vi "ecg_ncs_v5.vi"() -> ()   [LabVIEW 2016]
uses:
  <instrlib>/niUSRP/niUSRP Timestamp.ctl
  C:/Program Files/National Instruments/LabVIEW 2016/examples/Instrument IO/Serial/support/Serial - Settings.ctl
  State.ctl
  <vilib>/Instr/_visa.llb/VISA Configure Serial Port (Instr).vi
  <instrlib>/niUSRP/niUSRP Write Tx Data (2D CDB).vi
  <instrlib>/niUSRP/niUSRP Fetch Rx Data (2D CDB).vi
panel:
  in  "File Name 2":string="Test"
  in  "Path 2":path=path "D:/Research/SummerFall17Spring18/CnC/NCS/EcgNcsCorrelation/Labview Codes/ECG_NCS"
  out "#Loop = #Packets Received":i32
  out "ECGsample":i16
  out "PhNcs":dbl
  out "AmpNcs":dbl
  out "AmpNcsDS":dbl
  out "PhNcsDS":dbl
  out "error IO 2":errorcluster={"status"=FALSE, "code"=-1074118647, "source"=""}
  in  "Serial Settings":T1={"baud rate"=57600, "data bits"=8, "parity"=enum."None", "stop bits"=10, "flow control"=0} {"flow control" items=["None"=0, "XON/XOFF"=1, "RTS/CTS"=2, "DTR/DSR"=4]; "stop bits" items=["1.0"=10, "1.5"=15, "2.0"=20]; "data bits" min=5 max=8 step=1; "baud rate" items=["75"=75, "110"=110, "134"=134, "150"=150, "300"=300, "600"=600, "1200"=1200, "1800"=1800, "2400"=2400, "4800"=4800, "7200"=7200, "9600"=9600, "14400"=14400, "19200"=19200, "28800"=28800, "38400"=38400, "56000"=56000, "57600"=57600, "115200"=115200, "128000"=128000, "230400"=230400]}
  in  "VISA resource name":refnum<visa-resource-name>="bmd101"
  out "ECG":i16(graph)
  in  "byte count":u32=1
  out "Coerced Rx IQ Rate":dbl
  in  "Sampling Rate":i32=500
  out "Gain":dbl=-15.0
  out "Bandwidth":dbl=56000000.0
  out "Coerced Carrier Frequency":dbl=2000000000.0 format="%#.17g"
  out "Coerced Tx IQ rate":dbl=1000000.0
  out "error IO":errorcluster={"status"=FALSE, "code"=-1074118647, "source"=""}
  in  "Rx Number of Samples":i32=10000
  in  "Tab Control 2":enum32{"NI-294x/295x", "NI-2900/2901"}(tab)=enum."NI-2900/2901"
  in  "Rx carrier frequency [Hz]":dbl=2000000000.0 format="%#_6p"
  in  "Tx carrier frequency [Hz]":dbl=1000000000.0 format="%#_6p"
  in  "Start Trigger Time":T2={"whole seconds"=1, "fractional seconds"=0.0}
  in  "Tab Control":T3(tab)
  out "NCS tag Amp":dbl[](graph)=[0.011967714738528729, 0.012021355192189592, 0.012015275039596582, 0.011969166030167903, 0.011958890166168242, 0.012007893820858737, 0.012022893722444085, 0.011978222225113794, 0.011969989939463181, 0.012003099640895068]
  out "NCS tag Phase":dbl[](graph)=[0.011967714738528729, 0.012021355192189592, 0.012015275039596582, 0.011969166030167903, 0.011958890166168242, 0.012007893820858737, 0.012022893722444085, 0.011978222225113794, 0.011969989939463181, 0.012003099640895068]
  out "Tag Amp":dbl[](graph)
  out "Tag Phase":dbl[](graph)
  out "Tx Waveform Graph":waveform(dbl)[](graph)
  in  "Stop":bool
  in  "Channel 0\nTone Amplitude":dbl=0.707 step=0.05 format="%#.6g"
  in  "Channel 0 \nTone Frequency":dbl=5000.0 format="%#_6p"
  in  "Tx Waveform Size":dbl=2000.0
  in  "Device Name":refnum<k15>="MyB200"
  in  "Tx Gain":dbl=28.0 format="%#_6f"
  in  "Tx IQ Rate":dbl=1000000.0 format="%#_6p"
  in  "Rx Gain":dbl=32.0 format="%#_6f"
  in  "Rx IQ Rate":dbl=1000000.0 format="%#_6p"
  # "Rx Settings"
  # "Tx Settings"
  # "Note that on the NI-2900 and NI-2901, both Rx channels share an LO and both Tx channels share an LO. However, on the NI-294x/295x devices, Rx and Tx of channel 0 share an LO and Rx and Tx of channel 1 share an LO."
  # "Rx: Number of samples should be 1e6/512 in one loop."
  # "This Tx graph should always have end and start tied up since this is being sent in a loop continuously. Otherwise phase jumps will be noticed."
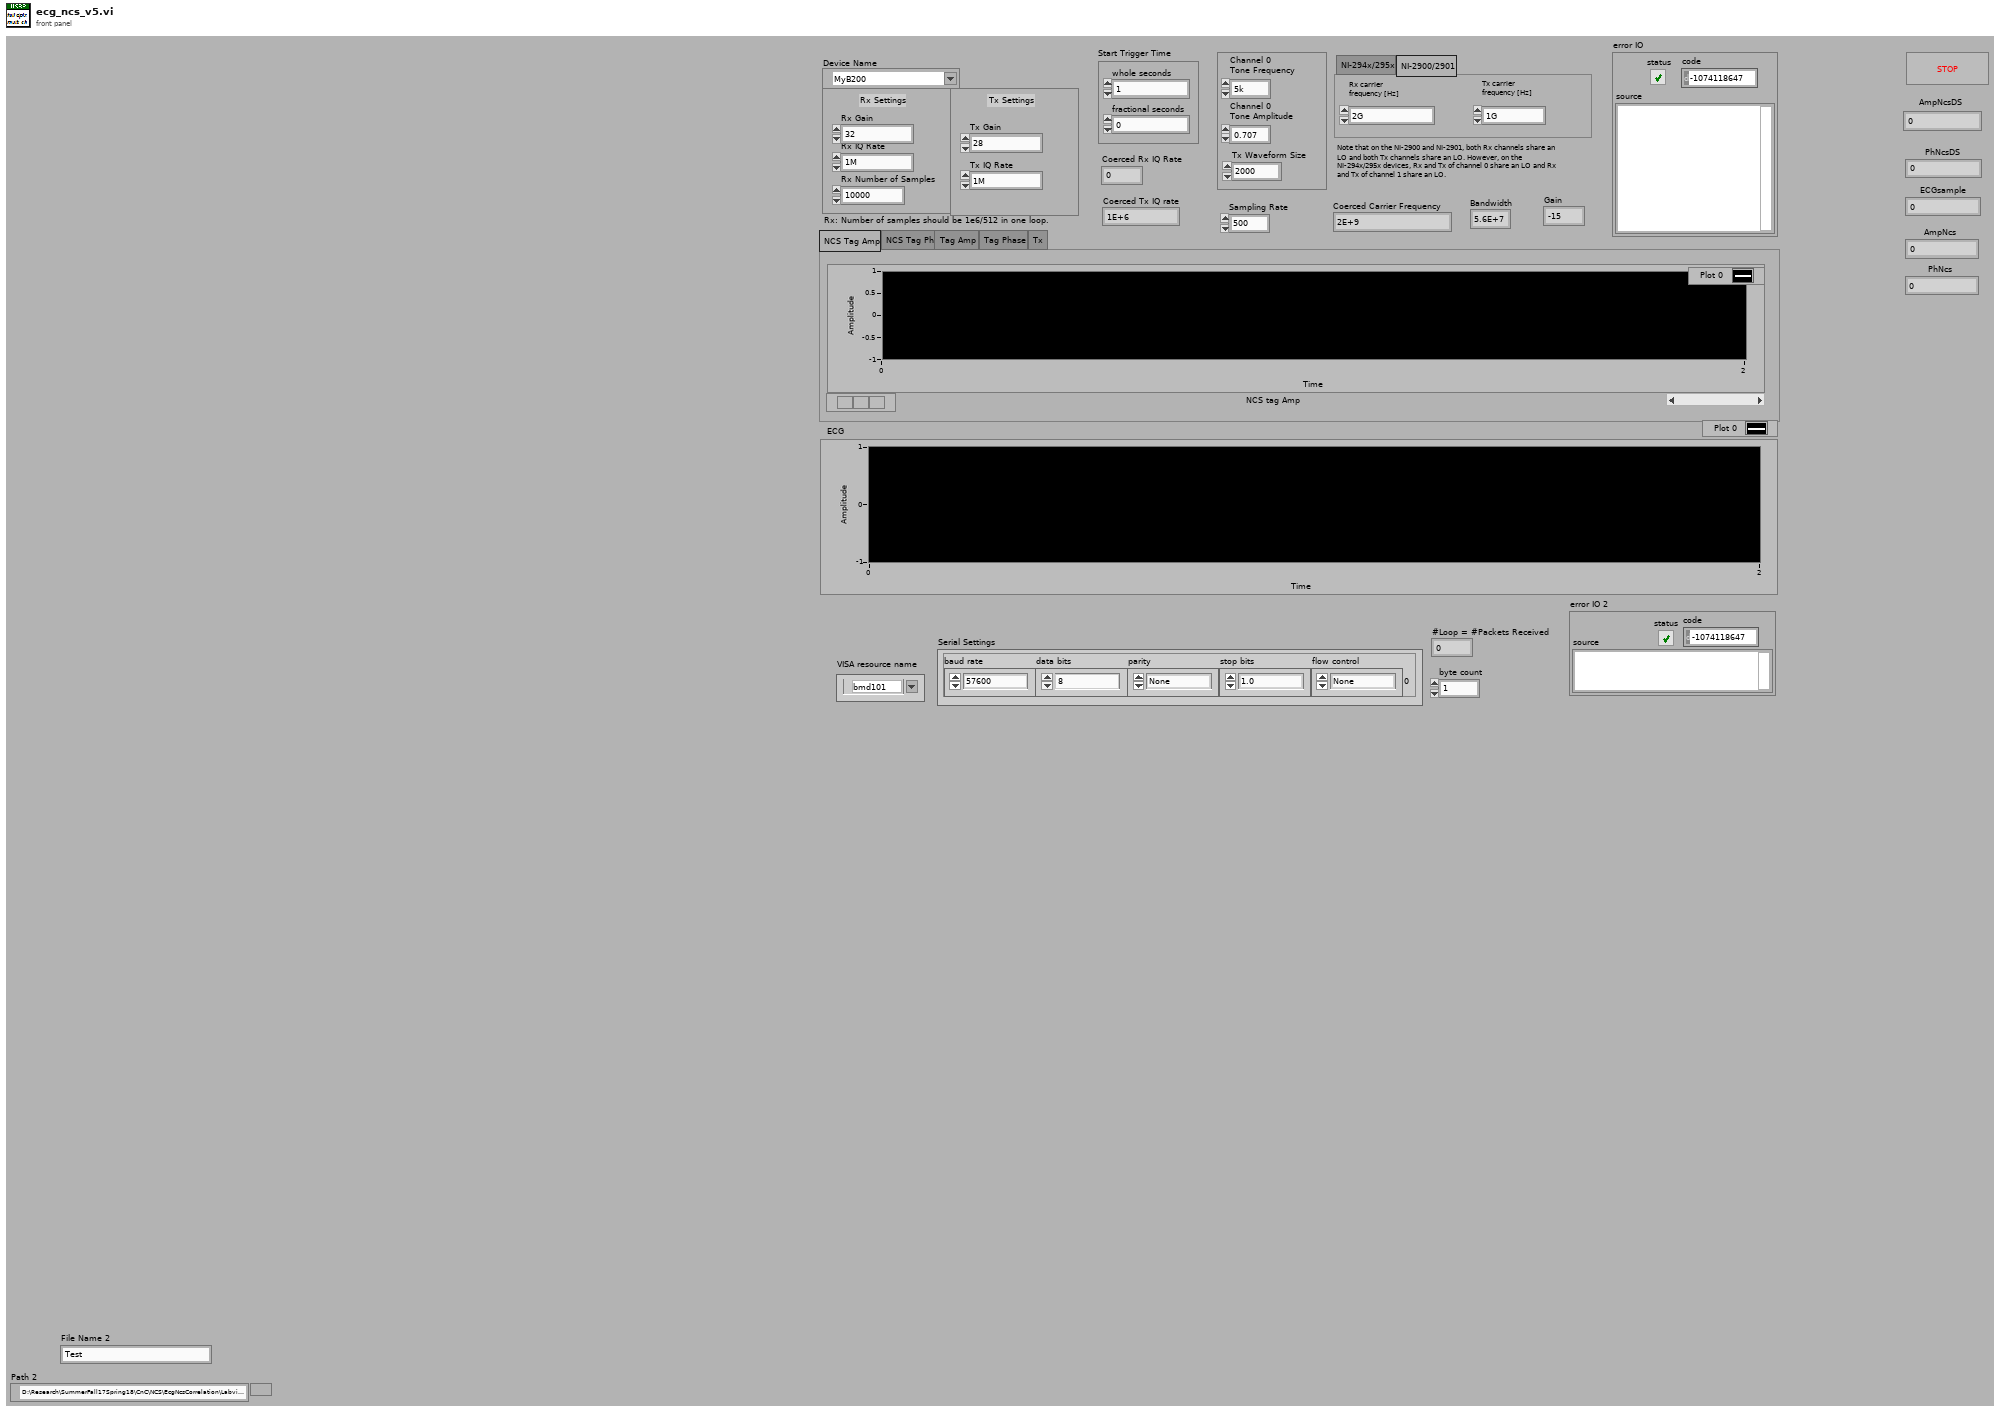
[diagram p1: front panel]
types:
  T1 = typedef "Serial - Settings.ctl" = cluster{"baud rate":u32, "data bits":u16, "parity":enum16{"None", "Odd", "Even", "Mark", "Space"}, "stop bits":u16, "flow control":u16}
  T2 = typedef "niUSRP Timestamp.ctl" = cluster{"whole seconds":u64, "fractional seconds":dbl}
  T3 = enum32{"NCS Tag Amp", "NCS Tag Ph", "Tag Amp", "Tag Phase", "Tx"}
  T4 = typedef "State.ctl" = enum16{"Initialize", "get byte", "check", "packet received", "packet approved"}
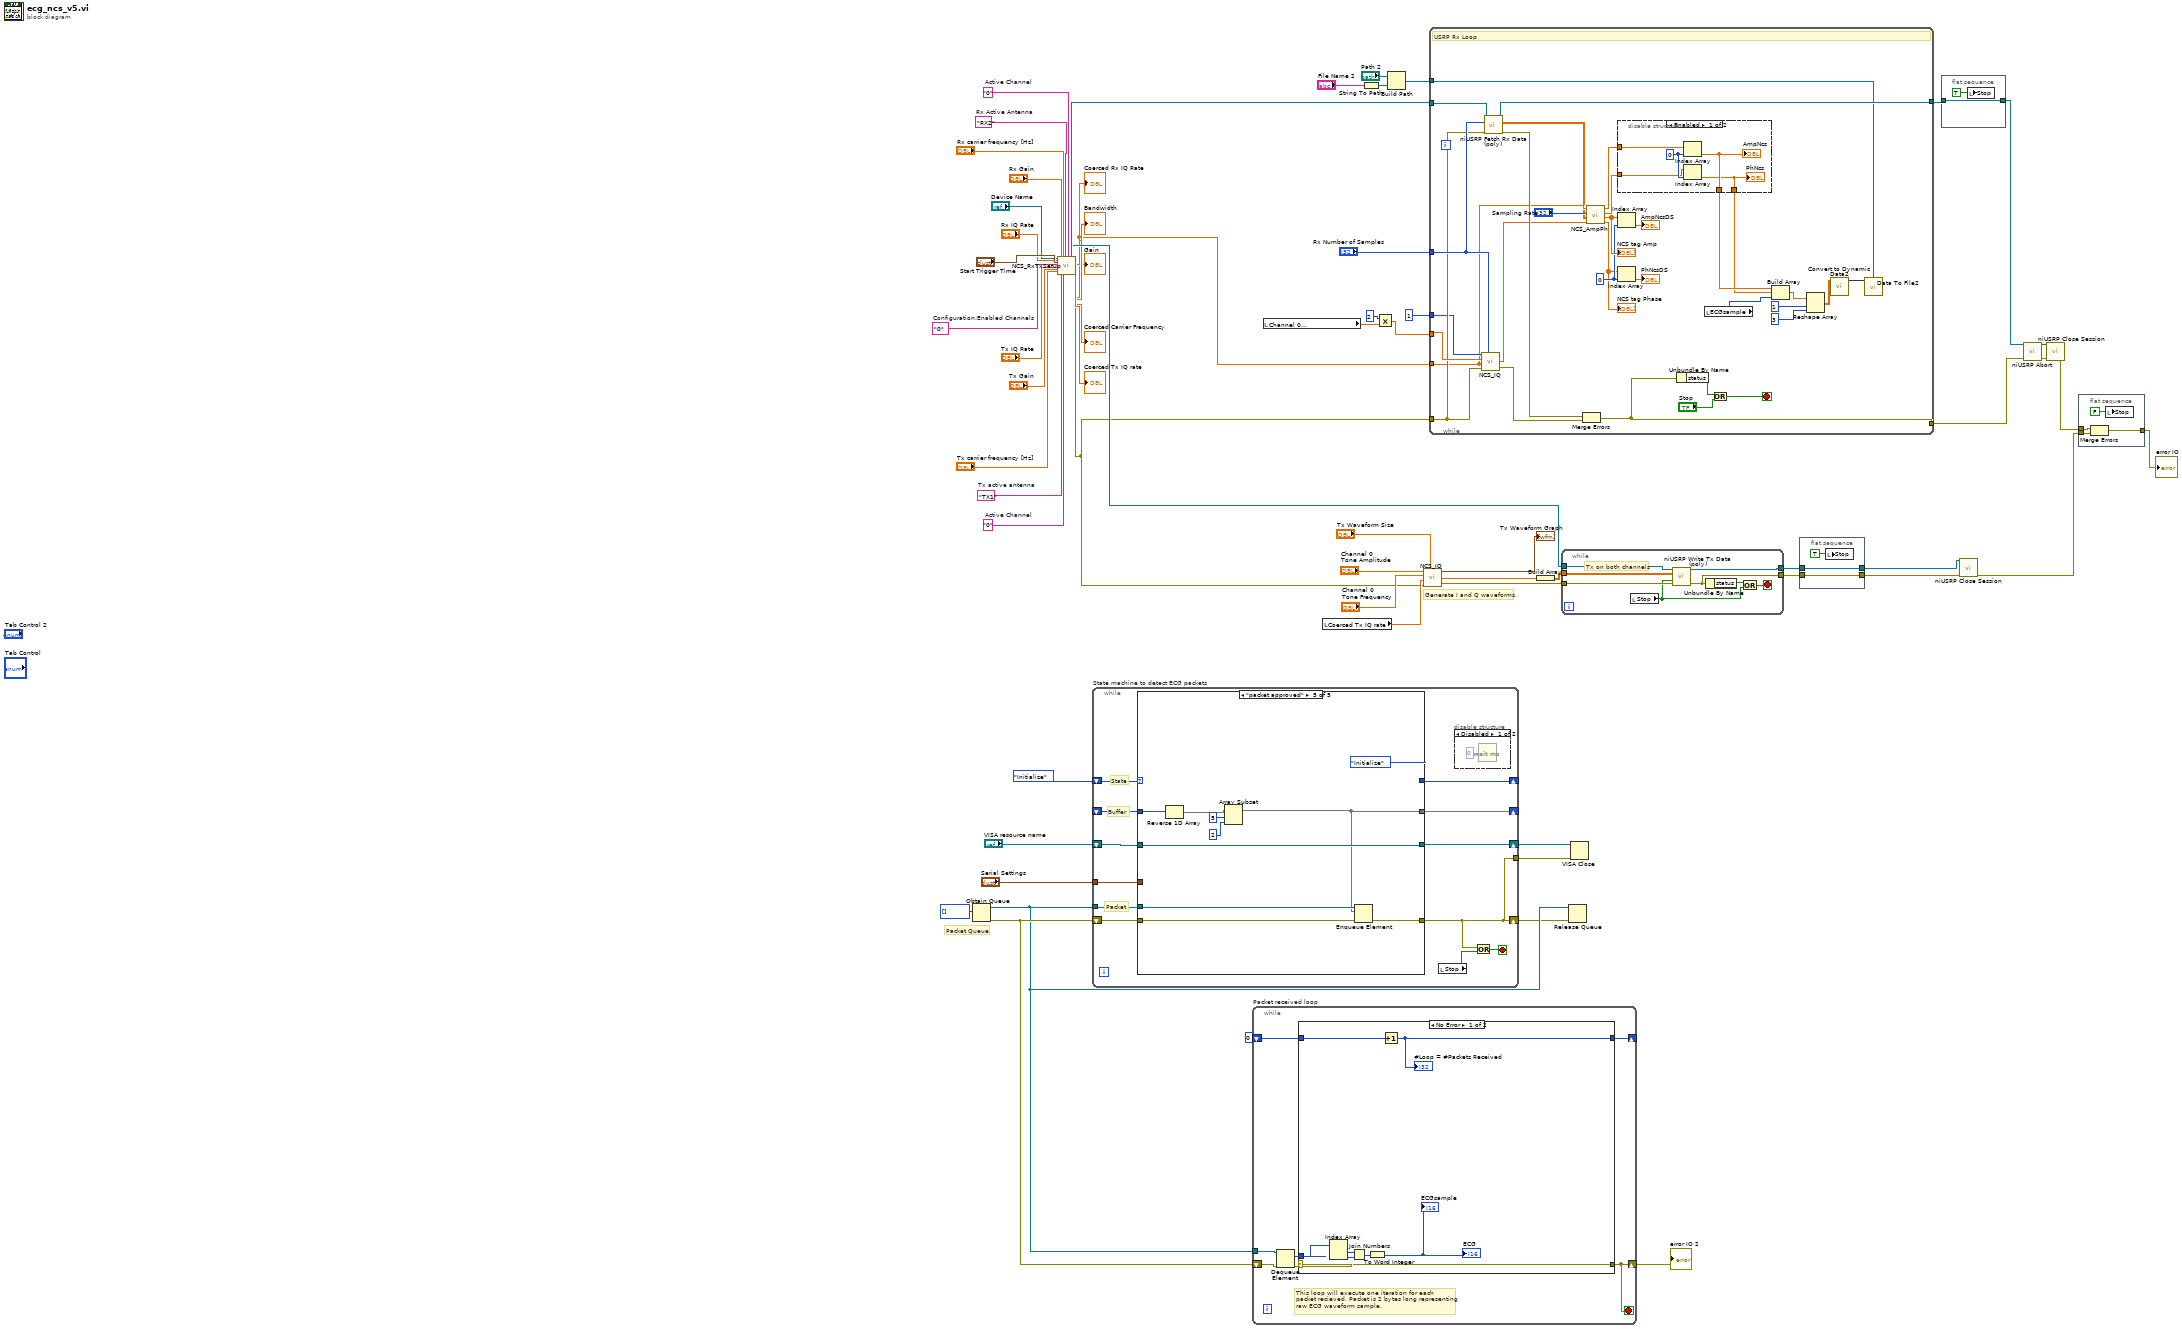
[diagram p0: block diagram]
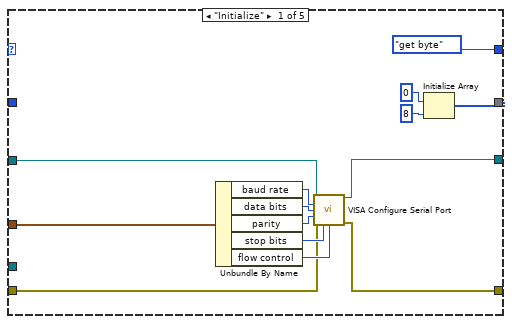
[diagram p4: hidden frame]
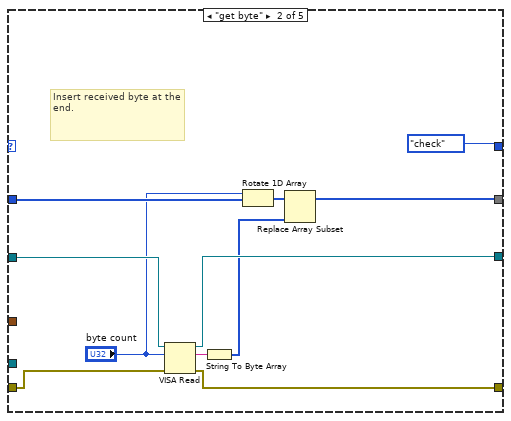
[diagram p5: hidden frame]
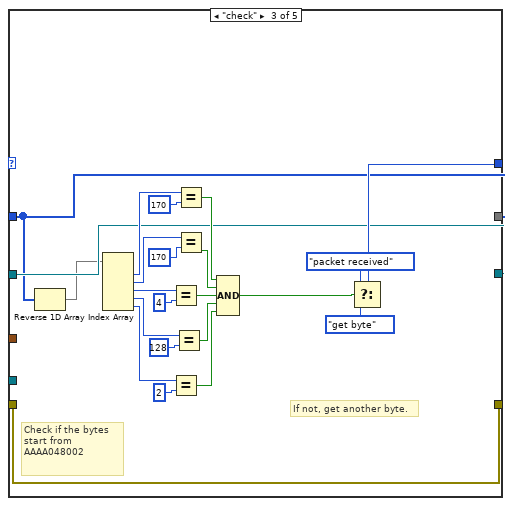
[diagram p6: hidden frame]
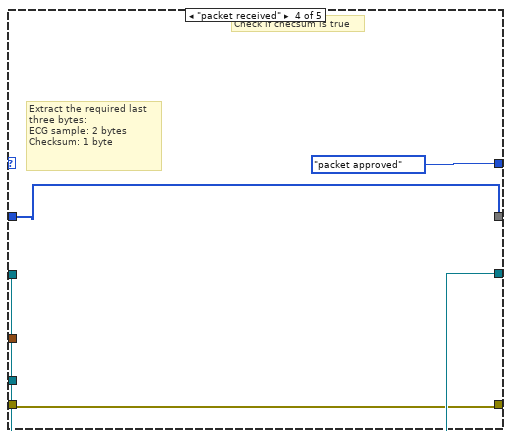
[diagram p7: hidden frame]
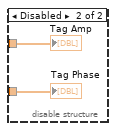
[diagram p8: hidden frame]
diagram:
  w17 = "0"  # Active Channel
  w18 = "0"  # Active Channel
  w53 = "RX2"  # Rx Active Antenna
  w49 = "TX1"  # Tx active antenna
  w35 = "0"  # Configuration:Enabled Channels
  # "Packet Queue"
  # "Generate I and Q waveforms."
  n1 = Obtain Queue(element data type=u8[] []) -> (queue out=w12:refnum<queue>, error out=w13:errorcluster)  [unwired: 4 in, 1 out]
  n2 = call "NCS_RxTxSetup.vi"("IVI Refnum in"="Device Name", "Rx IQ Rate"="Rx IQ Rate", "Start Trigger Time"="Start Trigger Time", "Configuration:Enabled Channels"=w35, "Tx IQ Rate"="Tx IQ Rate", "Tx Gain"="Tx Gain", "Tx carrier frequency [Hz]"="Tx carrier frequency [Hz]", "Rx Gain"="Rx Gain", "Tx active antenna"=w49, "Rx carrier frequency [Hz]"="Rx carrier frequency [Hz]", "Active Channel"=w17, "Rx Active Antenna"=w53, "Active Channel 2"=w18) -> ("session handle out"=w60:refnum<k15>, "IVI Refnum out"=w61:refnum<k15>, "Coerced Rx IQ Rate"=w16:dbl, "Bandwidth"=→"Bandwidth":dbl, "Gain"=→"Gain":dbl, "Carrier Frequency"=→"Coerced Carrier Frequency":dbl, "IQ Rate 2"=→"Coerced Tx IQ rate":dbl, "error out"=w28:errorcluster)  [unwired: 7 in]
  "Coerced Rx IQ Rate" <- w16
  n3 = while "State machine to detect ECG packets" {
    shift-right: [w64] -> w7
    shift-left: w13 -> [w70]
    shift-right: [w73] -> _
    shift-left: State."Initialize" ("State") -> [w72]
    shift-right: [w69] -> _
    shift-left: _ -> [w71]
    tunnel: w12 -> [w68]
    shift-right: [w67] -> w8
    shift-left: "VISA resource name" -> [w66]
    tunnel: "Serial Settings" -> [w65]
    tunnel: [w64] -> w6
    stop <- w63 stop-if-true
    # "State"
    # "Buffer"
    # "Packet"
    n4 = case shown="\"packet approved\"" w72 {
      tunnel: [w85 w97 w101 w124 w127] -> w69
      tunnel: [State."get byte" ("State") State."check" ("f") w121 State."packet approved" ("State") State."Initialize" ("State")] -> w73
      tunnel: w71 -> [_ w90 w101 w124 w129]
      tunnel: w70 -> [w79 w94 w122 w125 w132]
      tunnel: [w78 w93 w122 w125 w131] -> w64
      tunnel: w68 -> [_ _ _ _ w133]
      tunnel: [w77 w95 w102 w126 w130] -> w67
      tunnel: w66 -> [w76 w96 w102 w126 w130]
      tunnel: w65 -> [w75 _ _ _ _]
      frame "Initialize" {
        n5 = Unbundle By Name(w75) -> ("baud rate"=w84:u32, "data bits"=w83:u16, "parity"=w82:enum16{"None", "Odd", "Even", "Mark", "Space"}, "stop bits"=w81:u16, "flow control"=w80:u16)
        n6 = call-poly "VISA Configure Serial Port"("VISA resource name"=w76, "baud rate (9600)"=w84, "data bits (8)"=w83, "parity (0:none)"=w82, "error in (no error)"=w79, "stop bits (10: 1 bit)"=w81, "flow control (0:none)"=w80) -> ("VISA resource name out"=w77:refnum<visa-resource-name>, "error out"=w78:errorcluster)  [unwired: 3 in, 4 out]
        n7 = Initialize Array(u8 0, 8 ("dimension size")) -> (w85:u8[])
      }
      frame "get byte" {
        # "Insert received byte at the end."
        n8 = VISA Read(VISA resource name=w96, byte count="byte count", error in (no error)=w94) -> (VISA resource name out=w95:refnum<visa-resource-name>, read buffer=w92:string, error out=w93:errorcluster)  [unwired: 1 out]
        n9 = String To Byte Array(string=w92) -> (unsigned byte array=w91:u8[])
        n10 = Rotate 1D Array(1:w90, 2:"byte count") -> (0:w98:u8[])
        n11 = Replace Array Subset(array=w98, new element=w91) -> (w97:u8[])  [unwired: 1 in]
      }
      frame "check" {
        # "If not, get another byte."
        # "Check if the bytes start from AAAA048002"
        n12 = Reverse 1D Array(array=w101) -> (reversed array=w100:u8[])
        n13 = Index Array(array=w100) -> (element #1=w108:u8, element #2=w107:u8, element #3=w106:u8, element #4=w105:u8, element #5=w104:u8)  [unwired: 5 in]
        n14 = Equal?(x=w106, y=u8 4 ("element")) -> (x = y?=w111:bool)
        n15 = Equal?(x=w104, y=u8 2 ("element")) -> (x = y?=w109:bool)
        n16 = Equal?(x=w105, y=u8 128 ("element")) -> (x = y?=w110:bool)
        n17 = Equal?(x=w108, y=u8 170 ("element")) -> (x = y?=w113:bool)
        n18 = Equal?(x=w107, y=u8 170 ("element")) -> (x = y?=w112:bool)
        n19 = Compound Arithmetic op=AND(w113, w112, w111, w110, w109) -> (w103:bool)
        n20 = Select(t=State."packet received" ("f"), s=w103, f=State."get byte") -> (s? t:f=w121:T4)
      }
      frame "packet received" {
        # "Check if checsum is true"
        # "Extract the required last three bytes: \nECG sample: 2 bytes\nChecksum: 1 byte"
      }
      frame "packet approved" {
        n21 = Reverse 1D Array(array=w129) -> (reversed array=w128:u8[])
        n22 = Array Subset(array=w128, index=5, length=2 ("index")) -> (w127:u8[])
        n23 = Enqueue Element(queue=w133, element=w127, error in (no error)=w132) -> (error out=w131:errorcluster)  [unwired: 1 in, 2 out]
      }
    }
    n24 = local read "Stop"() -> (w62:bool)
    n25 = disable-structure shown="Disabled" {
      frame Disabled {
        n26 = Wait (ms)(milliseconds to wait=u32 0) -> ()  [unwired: 1 out]
      }
      frame Enabled {
      }
    }
    n27 = Or(x=w64, y=w62) -> (x .or. y?=w63:bool)
  }
  n28 = while "Packet received loop" {
    shift-right: [w139] -> w9
    shift-left: w13 -> [w143]
    tunnel: w12 -> [w142]
    shift-right: [w137] -> _
    shift-left: 0 -> [w138]
    stop <- w139 stop-if-true
    # "This loop will execute one iteration for each\npacket recieved. Packet is 2 bytes long representing \nraw ECG waveform sample."
    n29 = Dequeue Element(queue=w142, error in (no error)=w143) -> (element=w141:u8[], error out=w140:errorcluster)  [unwired: 1 in, 2 out]
    n30 = case shown="No Error" w140 {
      selector: w140 -> [w145 w153]
      tunnel: w141 -> [w151 _]
      tunnel: [w145 w153] -> w139
      tunnel: w138 -> [w147 w152]
      tunnel: [w146 w152] -> w137
      frame No Error {
        n31 = Index Array(array=w151) -> (element #1=w150:u8, element #2=w149:u8)  [unwired: 2 in]
        n32 = Join Numbers(hi=w150, lo=w149) -> ((hi.lo)=w148:u16)
        n33 = To Word Integer(number=w148) -> (16bit integer=→"ECG" →"ECGsample":i16)
        n34 = Increment(x=w147) -> (x+1=w146:i32)
        "#Loop = #Packets Received" <- w146
      }
      frame Error {
      }
    }
  }
  "error IO 2" <- w9
  n35 = local read "Channel 0 \nTone Frequency"() -> (w34:dbl)
  n36 = local read "Coerced Tx IQ rate"() -> (w29:dbl)
  n37 = String To Path(string="File Name 2") -> (path=w4:path)
  n38 = Multiply(x=2, y=w34) -> (x*y=w33:dbl)
  n39 = Build Path(base path="Path 2", name or relative path=w4) -> (appended path=w1:path)
  n40 = call "NCS_IQ.vi"("Tone Amplitude"="Channel 0\nTone Amplitude", "Waveform Size"="Tx Waveform Size", "Tone Frequency"="Channel 0 \nTone Frequency", "Coerced IQ rate"=w29, "error in (no error)"=w28) -> ("IQ waveform"=→"Tx Waveform Graph":waveform(dbl)[], "IQ waveform array"=w26:cdb[], "error out"=w27:errorcluster)  [unwired: 1 in]
  n41 = while {
    tunnel: w61 -> [w185]
    tunnel: w28 -> [w178]
    tunnel: [w184] -> w45
    tunnel: "Rx Number of Samples" -> [w180]
    tunnel: w16 -> [w174]
    tunnel: [w175] -> w37
    tunnel: w33 -> [w179]
    tunnel: 1 -> [w176]
    tunnel: w1 -> [w154]
    stop <- w181 stop-if-true
    w166 = 0
    # "USRP Rx Loop"
    n42 = call "NCS_IQ.vi"("Tone Amplitude"=w176, "Waveform Size"=w180, "Tone Frequency"=w179, "Coerced IQ rate"=w174, "error in (no error)"=w178) -> ("IQ waveform array"=w171:cdb[], "error out"=w177:errorcluster)  [unwired: 1 in, 1 out]
    n43 = call-poly <instrlib>:"niUSRP Fetch Rx Data (poly).vi"("session handle"=w185, "number of samples"=w180, "error in (no error)"=w178) -> ("session handle out"=w184:refnum<k15>, "data"=w172:cdb[][], "error out"=w182:errorcluster)  [unwired: 9 in, 1 out]
    n44 = Merge Errors(w182, w177) -> (w175:errorcluster)
    n45 = call "NCS_AmpPh.vi"("IQ"=w171, "data"=w172, "Sampling Rate"="Sampling Rate", "Coerced Rx IQ Rate"=w174) -> ("Phase DownSampled"=w165:dbl[], "Amp DownSampled"=w167:dbl[], "Phase"=w169:dbl[], "Amplitude"=w170:dbl[])  [unwired: 4 in]
    "NCS tag Amp" <- w167
    "NCS tag Phase" <- w165
    n46 = disable-structure shown="Enabled" {
      disable-tunnel: w170 -> [w189 w192]
      disable-tunnel: w169 -> [w188 w191]
      disable-tunnel: [w187 _] -> w156
      disable-tunnel: [w186 _] -> w155
      frame Enabled {
        w190 = 0
        n47 = Index Array(array=w189, index=w190) -> (element=w187:dbl)
        "AmpNcs" <- w187
        n48 = Index Array(array=w188, index=w190) -> (element=w186:dbl)
        "PhNcs" <- w186
      }
      frame Disabled {
        "Tag Amp" <- w192
        "Tag Phase" <- w191
      }
    }
    n49 = Index Array(array=w167, index=w166) -> (element=→"AmpNcsDS":dbl)
    n50 = Index Array(array=w165, index=w166) -> (element=→"PhNcsDS":dbl)
    n51 = Unbundle By Name(w175) -> ("status"=w183:bool)
    n52 = local read "ECGsample"() -> (w157:i16)
    n53 = Or(x=w183, y="Stop") -> (x .or. y?=w181:bool)
    n54 = Build Array(w156, w155, w157) -> (w161:dbl[])
    n55 = Reshape Array(w161, 1 ("dimension size"), 3 ("dimension size")) -> (w158:dbl[][])
    n56 = call "Convert to Dynamic Data2"("2D Array"=w158) -> ("Dynamic Data Type"=w162:dynamicdata)  [unwired: 3 in]
    n57 = call "Data To File2"("Signals"=w162, "Filename"=w154) -> ()  [unwired: 15 in, 3 out]
  }
  n58 = Build Array(w26) -> (w57:cdb[][])
  n59 = while {
    tunnel: w60 -> [w200]
    tunnel: w27 -> [w199]
    tunnel: [w197] -> w48
    tunnel: [w195] -> w43
    tunnel: w57 -> [w193]
    stop <- w196 stop-if-true
    # "Tx on both channels"
    n60 = local read "Stop"() -> (w194:bool)
    n61 = call-poly <instrlib>:"niUSRP Write Tx Data (poly).vi"("session handle"=w200, "data"=w193, "end of data?"=w194, "error in (no error)"=w199) -> ("session handle out"=w195:refnum<k15>, "error out"=w197:errorcluster)  [unwired: 10 in]
    n62 = Unbundle By Name(w197) -> ("status"=w198:bool)
    n63 = Compound Arithmetic op=OR(w198, w194) -> (w196:bool)
  }
  n64 = Release Queue(queue=w12, error in (no error)=w7) -> ()  [unwired: 1 in, 3 out]
  n65 = VISA Close(VISA resource name=w8, error in (no error)=w6) -> ()  [unwired: 1 out]
  n66 = flat-sequence {
    tunnel: [w202] -> w47
    tunnel: w48 -> [w202]
    tunnel: [w201] -> w44
    tunnel: w43 -> [w201]
    frame #0 {
      n67 = local write "Stop"(TRUE ("STOP")) -> ()
    }
  }
  n68 = flat-sequence {
    tunnel: [w204] -> w46
    tunnel: w45 -> [w204]
    frame #0 {
      n69 = local write "Stop"(TRUE ("STOP")) -> ()
    }
  }
  n70 = call <instrlib>:"niUSRP Close Session.vi"("session handle"=w44, "error in (no error)"=w47) -> ("error out"=w42:errorcluster)  [unwired: 13 in]
  n71 = call <instrlib>:"niUSRP Abort.vi"("session handle"=w46, "error in (no error)"=w37) -> ("session handle out"=w59:refnum<k15>, "error out"=w58:errorcluster)  [unwired: 12 in]
  n72 = call <instrlib>:"niUSRP Close Session.vi"("session handle"=w59, "error in (no error)"=w58) -> ("error out"=w39:errorcluster)  [unwired: 13 in]
  n73 = flat-sequence {
    tunnel: w42 -> [w208]
    tunnel: [w207] -> w40
    tunnel: w39 -> [w206]
    frame #0 {
      n74 = Merge Errors(w206, w208) -> (w207:errorcluster)
      n75 = local write "Stop"(FALSE ("STOP")) -> ()
    }
  }
  "error IO" <- w40
